vi "Untitled 5.vi"(8 "error in (no error)":errorcluster, 11 "Digital Reader in":refnum<class "Digital Reader.lvclass">) -> (0 "error out":errorcluster, 3 "Digital Reader out":refnum<class "Digital Reader.lvclass">)   [LabVIEW 2024]
uses:
  Digital Reader.lvclass/Digital Reader.ctl
  <vilib>/DAQmx/read.llb/DAQmx Read (Analog DBL 1Chan 1Samp).vi
  Digital Reader.lvclass
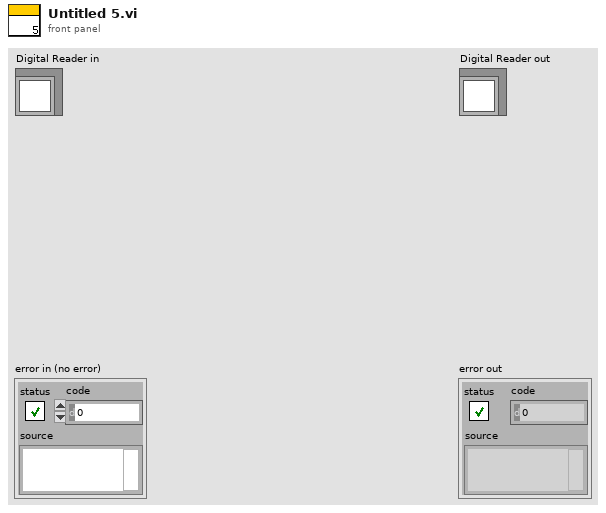
[diagram p1: front panel]
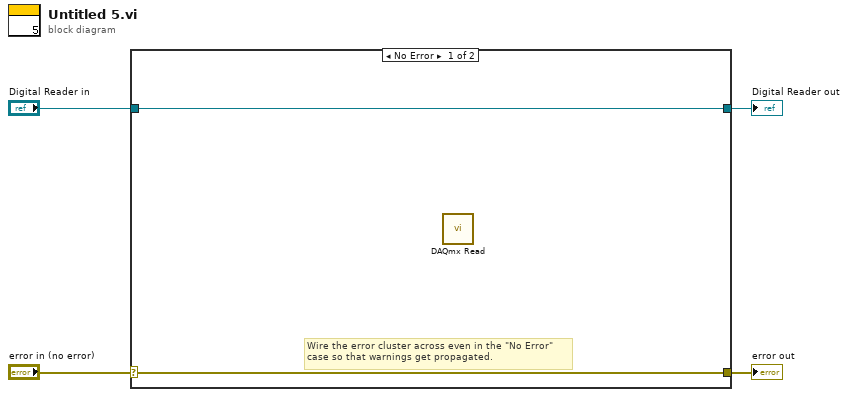
[diagram p0: block diagram]
diagram:
  n1 = case shown="No Error" "error in (no error)" {
    selector: "error in (no error)" -> [w5 w8]
    tunnel: [w5 w8] -> w3
    tunnel: [w6 w7] -> w1
    tunnel: "Digital Reader in" -> [w6 w7]
    frame No Error {
      # "Wire the error cluster across even in the \"No Error\"\ncase so that warnings get propagated."
      n2 = call-poly <vilib>:"DAQmx Read.vi"() -> ()  [unwired: 13 in, 3 out]
    }
    frame Error {
    }
  }
  "error out" <- w3
  "Digital Reader out" <- w1
